vi "QI_OpenLib.vi"(2 "error in (no error)":errorcluster, 3 "path to dll":path) -> (0 "error out":errorcluster, 1 "LibOpen error":i32)   [LabVIEW 2014]
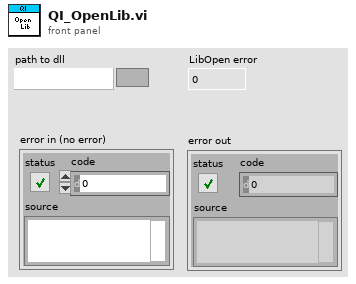
[diagram p1: front panel]
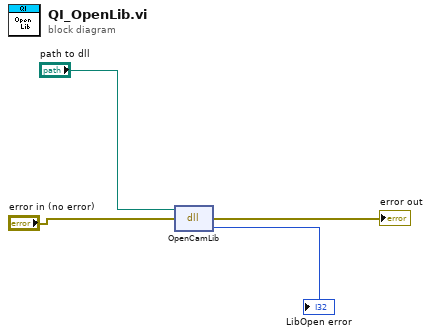
[diagram p0: block diagram]
diagram:
  n1 = dll-call lib="C:/Users/appli/Documents/Aline/octo-labview/QImaging/Release/QImaging.dll" fn="OpenCamLib"(path in="path to dll", error in="error in (no error)") -> (error out=→"error out":errorcluster, "return type"=→"LibOpen error":i32)  [unwired: 1 in, 1 out]
